vi "Init.vi"(8 "error in (no error)":errorcluster, 11 "rotator driver in":refnum<class "rotator driver.lvclass">) -> (0 "error out":errorcluster, 2 "Init Result":refnum<class "Acquired Result.lvclass">, 3 "rotator driver out":refnum<class "rotator driver.lvclass">)   [LabVIEW 2018, in "rotator driver.lvclass"]
uses:
  rotator driver.lvclass
  NHMFL_Core/Libraries/Instruments/Results/Acquired Result/Acquired Result.lvclass
  NHMFL_Core/Libraries/Instruments/Simple VISA Reader/Simple VISA Reader Driver.lvclass
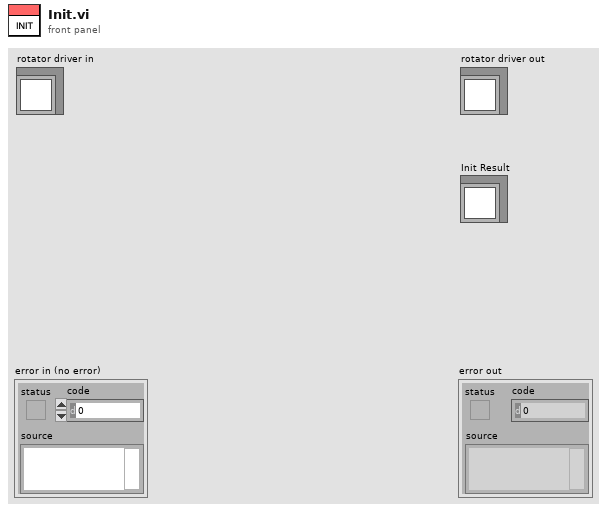
[diagram p1: front panel]
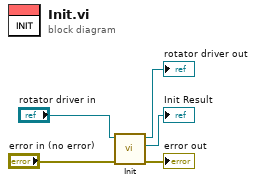
[diagram p0: block diagram]
diagram:
  n1 = call-parent "Init.vi"("error in (no error)"="error in (no error)", "Instrument Driver in"="rotator driver in") -> ("error out"=→"error out":errorcluster, "Init Result"=→"Init Result":refnum<class "Acquired Result.lvclass">, "Instrument Driver out"=→"rotator driver out":refnum<class "rotator driver.lvclass">)  [unwired: 7 in]
